vi "_Lock Server Down.vi"(4 "error in":errorcluster, 7 "Locked Ref":refnum<vi>) -> (0 "error out":errorcluster, 2 "Locked":bool)   [LabVIEW 2012]
uses:
  Type/_Server Control Type.ctl
panel:
  # "It takes normally 10-15 ms to complete"
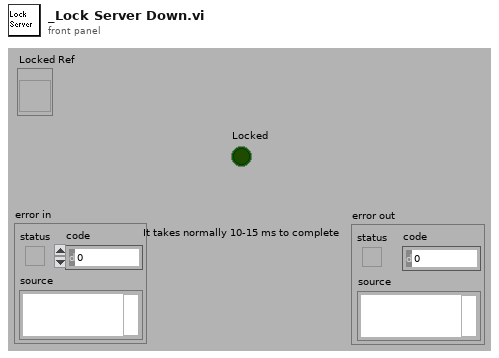
[diagram p1: front panel]
types:
  T1 = typedef "_Server Control Type.ctl" = enum16{"Command", "Boolean", "Text"}
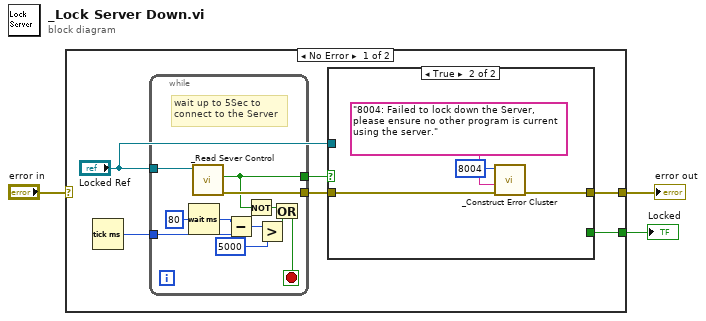
[diagram p0: block diagram]
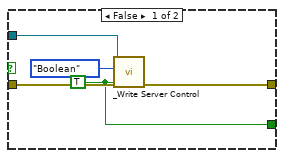
[diagram p2: hidden frame]
diagram:
  n1 = case shown="No Error" "error in" {
    selector: "error in" -> [_ w30]
    tunnel: [w6 w30] -> w3
    tunnel: [w5 _] -> w1
    frame No Error {
      n2 = Tick Count (ms)() -> (millisecond timer value=w4:u32)
      n3 = while {
        tunnel: [w20] -> w9
        tunnel: [w13] -> w8
        tunnel: "Locked Ref" -> [w19]
        tunnel: w4 -> [w16]
        stop <- w10 stop-if-true
        # "wait up to 5Sec to\nconnect to the Server"
        n4 = Wait (ms)(milliseconds to wait=u32 80) -> (millisecond timer value=w17:u32)
        n5 = call "_Read Sever Control.vi"("Control Ref"=w19) -> ("error out"=w20:errorcluster, "Boolean"=w13:bool)  [unwired: 2 in, 3 out]
        n6 = Subtract(x=w17, y=w16) -> (x-y=w15:u32)
        n7 = Not(x=w13) -> (.not. x?=w12:bool)
        n8 = Greater?(x=w15, y=u32 5000) -> (0:w11:bool)
        n9 = Or(x=w12, y=w11) -> (x .or. y?=w10:bool)
      }
      n10 = case shown="True" w8 {
        tunnel: w9 -> [w25 w28]
        tunnel: [w22 w27] -> w6
        tunnel: "Locked Ref" -> [w24 _]
        tunnel: [w21 _] -> w5
        frame False {
          w21 = TRUE ("Boolean (F)")
          n11 = call "_Write Server Control.vi"("error in (no error)"=w25, "Boolean (F)"=w21, "Control Type"=_Server_Control_Type."Boolean", "Control Ref"=w24) -> ("error out"=w22:errorcluster)  [unwired: 2 in, 3 out]
        }
        frame True {
          n12 = call "_Construct Error Cluster.vi"("error in"=w28, "reason"="8004: Failed to lock down the Server, please ensure no other program is current using the server." ("f"), "errorCode"=8004) -> ("error out"=w27:errorcluster)  [unwired: 1 in, 3 out]
        }
      }
    }
    frame Error {
    }
  }
  "error out" <- w3
  "Locked" <- w1
